vi "Lab Panel V4.87.vi"() -> ()   [LabVIEW 2013] (continued)
                      frame "CYCLE TEST" {
                      }
                      frame "T-RISE TEST" {
                      }
                    }
                    n1119 = Increment(x=w2157) -> (x+1=w2158:dbl)
                    n1120 = Greater Or Equal?(x=w2165, y=w2158) -> (x >= y?=w2167:bool)
                    n1121 = case shown="True" w2167 {
                      tunnel: w2162 -> [w2177 _]
                      tunnel: w2161 -> [w2176 _]
                      tunnel: w2160 -> [w2175 _]
                      tunnel: w2159 -> [w2174 _]
                      frame True {
                        n1122 = stacked-sequence {
                          tunnel: w2177 -> [w2181 _]
                          tunnel: w2176 -> [w2179 w2185]
                          tunnel: w2175 -> [_ w2188]
                          tunnel: w2174 -> [w2178 _]
                          frame #0 {
                            n1123 = Build Array(w2179) -> (w2182:string[])
                            n1124 = Build Array(w2181) -> (w2180:dbl[])
                            n1125 = TDMS Write(0:w2178, 5:"TEST PASS", 7:w2182, 9:w2180) -> (15:w2184:errorcluster)  [unwired: 2 in, 3 out]
                            n1126 = local write "data file error"(w2184) -> ()
                          }
                          frame #1 {
                            n1127 = Bundle(cluster=w2188, "STATUS"=w2185) -> (w2186:T4)  [unwired: 2 in]
                            n1128 = local write "RESULT LAB02-2"(TRUE) -> ()
                            n1129 = local write "DISP LAB02-2"(w2186) -> ()
                          }
                        }
                      }
                      frame False {
                      }
                    }
                  }
                }
              }
              frame #4 {
                # "LAB03-1"
                n1130 = Less?(x=w2189, y=2) -> (x < y?=w2192:bool)
                n1131 = local read "DISP LAB03-1"() -> (w2194:T4)
                n1132 = Unbundle(w2194) -> ("STATUS"=w2195:string)  [unwired: 2 out]
                n1133 = Equal?(x=w2195, y="RUN") -> (x = y?=w2191:bool)
                n1134 = And(x=w2191, y=w2192) -> (x .and. y?=w2190:bool)
                n1135 = case shown="True" w2190 {
                  tunnel: w2194 -> [_ w2200]
                  tunnel: w2189 -> [_ w2204]
                  frame False {
                  }
                  frame True {
                    n1136 = local read "SET LAB03-1"() -> (w2206:T5)
                    n1137 = local read "TDMS LAB03-1"() -> (w2199:refnum<k34>)
                    n1138 = Unbundle(w2200) -> ("CYCLE"=w2205:dbl)  [unwired: 2 out]
                    n1139 = Unbundle(w2206) -> ("CYCLES"=w2197:dbl, "T-RISE mins"=w2203:dbl)  [unwired: 3 out]
                    n1140 = case shown="\"T-RISE TEST\"" w2204 {
                      tunnel: w2203 -> [_ _ w2213]
                      tunnel: [w2208 w2210 w2213] -> w2202
                      tunnel: w2197 -> [w2208 w2210 _]
                      tunnel: ["CHART PASS" "CYCLE PASS" "T-RISE PASS"] -> w2201
                      frame "CHART TEST", Default {
                      }
                      frame "CYCLE TEST" {
                      }
                      frame "T-RISE TEST" {
                      }
                    }
                    n1141 = Increment(x=w2197) -> (x+1=w2198:dbl)
                    n1142 = Greater Or Equal?(x=w2205, y=w2198) -> (x >= y?=w2207:bool)
                    n1143 = case shown="True" w2207 {
                      tunnel: w2202 -> [w2217 _]
                      tunnel: w2201 -> [w2216 _]
                      tunnel: w2200 -> [w2215 _]
                      tunnel: w2199 -> [w2214 _]
                      frame True {
                        n1144 = stacked-sequence {
                          tunnel: w2217 -> [w2221 _]
                          tunnel: w2216 -> [w2219 w2225]
                          tunnel: w2215 -> [_ w2228]
                          tunnel: w2214 -> [w2218 _]
                          frame #0 {
                            n1145 = Build Array(w2219) -> (w2222:string[])
                            n1146 = Build Array(w2221) -> (w2220:dbl[])
                            n1147 = TDMS Write(0:w2218, 5:"TEST PASS", 7:w2222, 9:w2220) -> (15:w2224:errorcluster)  [unwired: 2 in, 3 out]
                            n1148 = local write "data file error"(w2224) -> ()
                          }
                          frame #1 {
                            n1149 = Bundle(cluster=w2228, "STATUS"=w2225) -> (w2226:T4)  [unwired: 2 in]
                            n1150 = local write "RESULT LAB03-1"(TRUE) -> ()
                            n1151 = local write "DISP LAB03-1"(w2226) -> ()
                          }
                        }
                      }
                      frame False {
                      }
                    }
                  }
                }
              }
              frame #5 {
                # "LAB03-2"
                n1152 = Less?(x=w2229, y=2) -> (x < y?=w2232:bool)
                n1153 = local read "DISP LAB03-2"() -> (w2234:T4)
                n1154 = Unbundle(w2234) -> ("STATUS"=w2235:string)  [unwired: 2 out]
                n1155 = Equal?(x=w2235, y="RUN") -> (x = y?=w2231:bool)
                n1156 = And(x=w2231, y=w2232) -> (x .and. y?=w2230:bool)
                n1157 = case shown="True" w2230 {
                  tunnel: w2234 -> [_ w2240]
                  tunnel: w2229 -> [_ w2244]
                  frame False {
                  }
                  frame True {
                    n1158 = local read "SET LAB03-2"() -> (w2246:T5)
                    n1159 = local read "TDMS LAB03-2"() -> (w2239:refnum<k34>)
                    n1160 = Unbundle(w2240) -> ("CYCLE"=w2245:dbl)  [unwired: 2 out]
                    n1161 = Unbundle(w2246) -> ("CYCLES"=w2237:dbl, "T-RISE mins"=w2243:dbl)  [unwired: 3 out]
                    n1162 = case shown="\"T-RISE TEST\"" w2244 {
                      tunnel: w2243 -> [_ _ w2253]
                      tunnel: [w2248 w2250 w2253] -> w2242
                      tunnel: w2237 -> [w2248 w2250 _]
                      tunnel: ["CHART PASS" "CYCLE PASS" "T-RISE PASS"] -> w2241
                      frame "CHART TEST", Default {
                      }
                      frame "CYCLE TEST" {
                      }
                      frame "T-RISE TEST" {
                      }
                    }
                    n1163 = Increment(x=w2237) -> (x+1=w2238:dbl)
                    n1164 = Greater Or Equal?(x=w2245, y=w2238) -> (x >= y?=w2247:bool)
                    n1165 = case shown="True" w2247 {
                      tunnel: w2242 -> [w2257 _]
                      tunnel: w2241 -> [w2256 _]
                      tunnel: w2240 -> [w2255 _]
                      tunnel: w2239 -> [w2254 _]
                      frame True {
                        n1166 = stacked-sequence {
                          tunnel: w2257 -> [w2261 _]
                          tunnel: w2256 -> [w2259 w2265]
                          tunnel: w2255 -> [_ w2268]
                          tunnel: w2254 -> [w2258 _]
                          frame #0 {
                            n1167 = Build Array(w2259) -> (w2262:string[])
                            n1168 = Build Array(w2261) -> (w2260:dbl[])
                            n1169 = TDMS Write(0:w2258, 5:"TEST PASS", 7:w2262, 9:w2260) -> (15:w2264:errorcluster)  [unwired: 2 in, 3 out]
                            n1170 = local write "data file error"(w2264) -> ()
                          }
                          frame #1 {
                            n1171 = Bundle(cluster=w2268, "STATUS"=w2265) -> (w2266:T4)  [unwired: 2 in]
                            n1172 = local write "RESULT LAB03-2"(TRUE) -> ()
                            n1173 = local write "DISP LAB03-2"(w2266) -> ()
                          }
                        }
                      }
                      frame False {
                      }
                    }
                  }
                }
              }
              frame #6 {
                # "LAB04-1"
                n1174 = Less?(x=w2269, y=2) -> (x < y?=w2272:bool)
                n1175 = local read "DISP LAB04-1"() -> (w2274:T4)
                n1176 = Unbundle(w2274) -> ("STATUS"=w2275:string)  [unwired: 2 out]
                n1177 = Equal?(x=w2275, y="RUN") -> (x = y?=w2271:bool)
                n1178 = And(x=w2271, y=w2272) -> (x .and. y?=w2270:bool)
                n1179 = case shown="True" w2270 {
                  tunnel: w2274 -> [_ w2280]
                  tunnel: w2269 -> [_ w2284]
                  frame False {
                  }
                  frame True {
                    n1180 = local read "SET LAB04-1"() -> (w2286:T5)
                    n1181 = local read "TDMS LAB04-1"() -> (w2279:refnum<k34>)
                    n1182 = Unbundle(w2280) -> ("CYCLE"=w2285:dbl)  [unwired: 2 out]
                    n1183 = Unbundle(w2286) -> ("CYCLES"=w2277:dbl, "T-RISE mins"=w2283:dbl)  [unwired: 3 out]
                    n1184 = case shown="\"T-RISE TEST\"" w2284 {
                      tunnel: w2283 -> [_ _ w2293]
                      tunnel: [w2288 w2290 w2293] -> w2282
                      tunnel: w2277 -> [w2288 w2290 _]
                      tunnel: ["CHART PASS" "CYCLE PASS" "T-RISE PASS"] -> w2281
                      frame "CHART TEST", Default {
                      }
                      frame "CYCLE TEST" {
                      }
                      frame "T-RISE TEST" {
                      }
                    }
                    n1185 = Increment(x=w2277) -> (x+1=w2278:dbl)
                    n1186 = Greater Or Equal?(x=w2285, y=w2278) -> (x >= y?=w2287:bool)
                    n1187 = case shown="True" w2287 {
                      tunnel: w2282 -> [w2297 _]
                      tunnel: w2281 -> [w2296 _]
                      tunnel: w2280 -> [w2295 _]
                      tunnel: w2279 -> [w2294 _]
                      frame True {
                        n1188 = stacked-sequence {
                          tunnel: w2297 -> [w2301 _]
                          tunnel: w2296 -> [w2299 w2305]
                          tunnel: w2295 -> [_ w2308]
                          tunnel: w2294 -> [w2298 _]
                          frame #0 {
                            n1189 = Build Array(w2299) -> (w2302:string[])
                            n1190 = Build Array(w2301) -> (w2300:dbl[])
                            n1191 = TDMS Write(0:w2298, 5:"TEST PASS", 7:w2302, 9:w2300) -> (15:w2304:errorcluster)  [unwired: 2 in, 3 out]
                            n1192 = local write "data file error"(w2304) -> ()
                          }
                          frame #1 {
                            n1193 = Bundle(cluster=w2308, "STATUS"=w2305) -> (w2306:T4)  [unwired: 2 in]
                            n1194 = local write "RESULT LAB04-1"(TRUE) -> ()
                            n1195 = local write "DISP LAB04-1"(w2306) -> ()
                          }
                        }
                      }
                      frame False {
                      }
                    }
                  }
                }
              }
              frame #7 {
                # "LAB04-2"
                n1196 = Less?(x=w2309, y=2) -> (x < y?=w2312:bool)
                n1197 = local read "DISP LAB04-2"() -> (w2314:T4)
                n1198 = Unbundle(w2314) -> ("STATUS"=w2315:string)  [unwired: 2 out]
                n1199 = Equal?(x=w2315, y="RUN") -> (x = y?=w2311:bool)
                n1200 = And(x=w2311, y=w2312) -> (x .and. y?=w2310:bool)
                n1201 = case shown="True" w2310 {
                  tunnel: w2314 -> [_ w2320]
                  tunnel: w2309 -> [_ w2324]
                  frame False {
                  }
                  frame True {
                    n1202 = local read "SET LAB04-2"() -> (w2326:T5)
                    n1203 = local read "TDMS LAB04-2"() -> (w2319:refnum<k34>)
                    n1204 = Unbundle(w2320) -> ("CYCLE"=w2325:dbl)  [unwired: 2 out]
                    n1205 = Unbundle(w2326) -> ("CYCLES"=w2317:dbl, "T-RISE mins"=w2323:dbl)  [unwired: 3 out]
                    n1206 = case shown="\"T-RISE TEST\"" w2324 {
                      tunnel: w2323 -> [_ _ w2333]
                      tunnel: [w2328 w2330 w2333] -> w2322
                      tunnel: w2317 -> [w2328 w2330 _]
                      tunnel: ["CHART PASS" "CYCLE PASS" "T-RISE PASS"] -> w2321
                      frame "CHART TEST", Default {
                      }
                      frame "CYCLE TEST" {
                      }
                      frame "T-RISE TEST" {
                      }
                    }
                    n1207 = Increment(x=w2317) -> (x+1=w2318:dbl)
                    n1208 = Greater Or Equal?(x=w2325, y=w2318) -> (x >= y?=w2327:bool)
                    n1209 = case shown="True" w2327 {
                      tunnel: w2322 -> [w2337 _]
                      tunnel: w2321 -> [w2336 _]
                      tunnel: w2320 -> [w2335 _]
                      tunnel: w2319 -> [w2334 _]
                      frame True {
                        n1210 = stacked-sequence {
                          tunnel: w2337 -> [w2341 _]
                          tunnel: w2336 -> [w2339 w2345]
                          tunnel: w2335 -> [_ w2348]
                          tunnel: w2334 -> [w2338 _]
                          frame #0 {
                            n1211 = Build Array(w2339) -> (w2342:string[])
                            n1212 = Build Array(w2341) -> (w2340:dbl[])
                            n1213 = TDMS Write(0:w2338, 5:"TEST PASS", 7:w2342, 9:w2340) -> (15:w2344:errorcluster)  [unwired: 2 in, 3 out]
                            n1214 = local write "data file error"(w2344) -> ()
                          }
                          frame #1 {
                            n1215 = Bundle(cluster=w2348, "STATUS"=w2345) -> (w2346:T4)  [unwired: 2 in]
                            n1216 = local write "RESULT LAB04-2"(TRUE) -> ()
                            n1217 = local write "DISP LAB04-2"(w2346) -> ()
                          }
                        }
                      }
                      frame False {
                      }
                    }
                  }
                }
              }
              frame #8 {
                # "LAB05-1"
                n1218 = Less?(x=w2349, y=2) -> (x < y?=w2352:bool)
                n1219 = local read "DISP LAB05-1"() -> (w2354:T4)
                n1220 = Unbundle(w2354) -> ("STATUS"=w2355:string)  [unwired: 2 out]
                n1221 = Equal?(x=w2355, y="RUN") -> (x = y?=w2351:bool)
                n1222 = And(x=w2351, y=w2352) -> (x .and. y?=w2350:bool)
                n1223 = case shown="True" w2350 {
                  tunnel: w2354 -> [_ w2360]
                  tunnel: w2349 -> [_ w2364]
                  frame False {
                  }
                  frame True {
                    n1224 = local read "SET LAB05-1"() -> (w2366:T5)
                    n1225 = local read "TDMS LAB05-1"() -> (w2359:refnum<k34>)
                    n1226 = Unbundle(w2360) -> ("CYCLE"=w2365:dbl)  [unwired: 2 out]
                    n1227 = Unbundle(w2366) -> ("CYCLES"=w2357:dbl, "T-RISE mins"=w2363:dbl)  [unwired: 3 out]
                    n1228 = case shown="\"T-RISE TEST\"" w2364 {
                      tunnel: w2363 -> [_ _ w2373]
                      tunnel: [w2368 w2370 w2373] -> w2362
                      tunnel: w2357 -> [w2368 w2370 _]
                      tunnel: ["CHART PASS" "CYCLE PASS" "T-RISE PASS"] -> w2361
                      frame "CHART TEST", Default {
                      }
                      frame "CYCLE TEST" {
                      }
                      frame "T-RISE TEST" {
                      }
                    }
                    n1229 = Increment(x=w2357) -> (x+1=w2358:dbl)
                    n1230 = Greater Or Equal?(x=w2365, y=w2358) -> (x >= y?=w2367:bool)
                    n1231 = case shown="True" w2367 {
                      tunnel: w2362 -> [w2377 _]
                      tunnel: w2361 -> [w2376 _]
                      tunnel: w2360 -> [w2375 _]
                      tunnel: w2359 -> [w2374 _]
                      frame True {
                        n1232 = stacked-sequence {
                          tunnel: w2377 -> [w2381 _]
                          tunnel: w2376 -> [w2379 w2385]
                          tunnel: w2375 -> [_ w2388]
                          tunnel: w2374 -> [w2378 _]
                          frame #0 {
                            n1233 = Build Array(w2379) -> (w2382:string[])
                            n1234 = Build Array(w2381) -> (w2380:dbl[])
                            n1235 = TDMS Write(0:w2378, 5:"TEST PASS", 7:w2382, 9:w2380) -> (15:w2384:errorcluster)  [unwired: 2 in, 3 out]
                            n1236 = local write "data file error"(w2384) -> ()
                          }
                          frame #1 {
                            n1237 = Bundle(cluster=w2388, "STATUS"=w2385) -> (w2386:T4)  [unwired: 2 in]
                            n1238 = local write "RESULT LAB05-1"(TRUE) -> ()
                            n1239 = local write "DISP LAB05-1"(w2386) -> ()
                          }
                        }
                      }
                      frame False {
                      }
                    }
                  }
                }
              }
              frame #9 {
                # "LAB05-2"
                n1240 = Less?(x=w2389, y=2) -> (x < y?=w2392:bool)
                n1241 = local read "DISP LAB05-2"() -> (w2394:T4)
                n1242 = Unbundle(w2394) -> ("STATUS"=w2395:string)  [unwired: 2 out]
                n1243 = Equal?(x=w2395, y="RUN") -> (x = y?=w2391:bool)
                n1244 = And(x=w2391, y=w2392) -> (x .and. y?=w2390:bool)
                n1245 = case shown="True" w2390 {
                  tunnel: w2394 -> [_ w2400]
                  tunnel: w2389 -> [_ w2404]
                  frame False {
                  }
                  frame True {
                    n1246 = local read "SET LAB05-2"() -> (w2406:T5)
                    n1247 = local read "TDMS LAB05-2"() -> (w2399:refnum<k34>)
                    n1248 = Unbundle(w2400) -> ("CYCLE"=w2405:dbl)  [unwired: 2 out]
                    n1249 = Unbundle(w2406) -> ("CYCLES"=w2397:dbl, "T-RISE mins"=w2403:dbl)  [unwired: 3 out]
                    n1250 = case shown="\"T-RISE TEST\"" w2404 {
                      tunnel: w2403 -> [_ _ w2413]
                      tunnel: [w2408 w2410 w2413] -> w2402
                      tunnel: w2397 -> [w2408 w2410 _]
                      tunnel: ["CHART PASS" "CYCLE PASS" "T-RISE PASS"] -> w2401
                      frame "CHART TEST", Default {
                      }
                      frame "CYCLE TEST" {
                      }
                      frame "T-RISE TEST" {
                      }
                    }
                    n1251 = Increment(x=w2397) -> (x+1=w2398:dbl)
                    n1252 = Greater Or Equal?(x=w2405, y=w2398) -> (x >= y?=w2407:bool)
                    n1253 = case shown="True" w2407 {
                      tunnel: w2402 -> [w2417 _]
                      tunnel: w2401 -> [w2416 _]
                      tunnel: w2400 -> [w2415 _]
                      tunnel: w2399 -> [w2414 _]
                      frame True {
                        n1254 = stacked-sequence {
                          tunnel: w2417 -> [w2421 _]
                          tunnel: w2416 -> [w2419 w2425]
                          tunnel: w2415 -> [_ w2428]
                          tunnel: w2414 -> [w2418 _]
                          frame #0 {
                            n1255 = Build Array(w2419) -> (w2422:string[])
                            n1256 = Build Array(w2421) -> (w2420:dbl[])
                            n1257 = TDMS Write(0:w2418, 5:"TEST PASS", 7:w2422, 9:w2420) -> (15:w2424:errorcluster)  [unwired: 2 in, 3 out]
                            n1258 = local write "data file error"(w2424) -> ()
                          }
                          frame #1 {
                            n1259 = Bundle(cluster=w2428, "STATUS"=w2425) -> (w2426:T4)  [unwired: 2 in]
                            n1260 = local write "RESULT LAB05-2"(TRUE) -> ()
                            n1261 = local write "DISP LAB05-2"(w2426) -> ()
                          }
                        }
                      }
                      frame False {
                      }
                    }
                  }
                }
              }
            }
          }
          frame #5 {
            # "check if test cycles reached for temperature rise test"
            n1262 = stacked-sequence {
              tunnel: w2458 -> [_ _ _ _ _ _ _ _ _ _]
              tunnel: w2457 -> [_ _ _ _ _ _ _ _ _ _]
              tunnel: w2456 -> [_ _ _ _ _ _ _ _ _ _]
              tunnel: w2455 -> [_ _ _ _ _ _ _ _ _ _]
              tunnel: w2454 -> [_ _ _ _ _ _ _ _ _ _]
              tunnel: w2453 -> [_ _ _ _ _ _ _ _ _ _]
              tunnel: w2452 -> [_ _ _ _ _ _ _ _ _ _]
              tunnel: w2451 -> [_ _ _ _ _ _ _ _ _ _]
              tunnel: w2450 -> [_ _ _ _ _ _ _ _ _ _]
              tunnel: w2449 -> [_ _ _ _ _ _ _ _ _ _]
              tunnel: w2448 -> [w2464 _ _ _ _ _ _ _ _ _]
              tunnel: w2438 -> [w2459 _ _ _ _ _ _ _ _ _]
              tunnel: w2447 -> [_ w2490 _ _ _ _ _ _ _ _]
              tunnel: w2446 -> [_ _ w2520 _ _ _ _ _ _ _]
              tunnel: w2445 -> [_ _ _ w2550 _ _ _ _ _ _]
              tunnel: w2444 -> [_ _ _ _ w2580 _ _ _ _ _]
              tunnel: w2443 -> [_ _ _ _ _ w2610 _ _ _ _]
              tunnel: w2442 -> [_ _ _ _ _ _ w2640 _ _ _]
              tunnel: w2441 -> [_ _ _ _ _ _ _ w2670 _ _]
              tunnel: w2440 -> [_ _ _ _ _ _ _ _ w2700 _]
              tunnel: w2439 -> [_ _ _ _ _ _ _ _ _ w2730]
              tunnel: w2437 -> [_ w2489 _ _ _ _ _ _ _ _]
              tunnel: w2436 -> [_ _ w2519 _ _ _ _ _ _ _]
              tunnel: w2435 -> [_ _ _ w2549 _ _ _ _ _ _]
              tunnel: w2434 -> [_ _ _ _ w2579 _ _ _ _ _]
              tunnel: w2433 -> [_ _ _ _ _ w2609 _ _ _ _]
              tunnel: w2432 -> [_ _ _ _ _ _ w2639 _ _ _]
              tunnel: w2431 -> [_ _ _ _ _ _ _ w2669 _ _]
              tunnel: w2430 -> [_ _ _ _ _ _ _ _ w2699 _]
              tunnel: w2429 -> [_ _ _ _ _ _ _ _ _ w2729]
              frame #0 {
                # "LAB01-1"
                n1263 = Equal?(x=w2464, y=2) -> (x = y?=w2462:bool)
                n1264 = local read "DISP LAB01-1"() -> (w2465:T4)
                n1265 = Unbundle(w2465) -> ("STATUS"=w2466:string)  [unwired: 2 out]
                n1266 = Equal?(x=w2466, y="RUN") -> (x = y?=w2461:bool)
                n1267 = And(x=w2461, y=w2462) -> (x .and. y?=w2460:bool)
                n1268 = case shown="True" w2460 {
                  tunnel: w2465 -> [_ w2469]
                  tunnel: w2459 -> [_ w2472]
                  frame False {
                  }
                  frame True {
                    n1269 = local read "SET LAB01-1"() -> (w2471:T5)
                    n1270 = local read "TDMS LAB01-1"() -> (w2468:refnum<k34>)
                    n1271 = Unbundle(w2469) -> ("CYCLE"=w2473:dbl)  [unwired: 2 out]
                    n1272 = Unbundle(w2471) -> ("T-RISE mins"=w2470:dbl)  [unwired: 4 out]
                    n1273 = Greater Or Equal?(x=w2473, y=w2472) -> (x >= y?=w2474:bool)
                    n1274 = case shown="True" w2474 {
                      tunnel: w2470 -> [w2477 _]
                      tunnel: w2469 -> [w2476 _]
                      tunnel: w2468 -> [w2475 _]
                      frame True {
                        n1275 = stacked-sequence {
                          tunnel: w2477 -> [w2480 _]
                          tunnel: w2476 -> [_ w2485]
                          tunnel: w2475 -> [w2478 _]
                          frame #0 {
                            n1276 = Build Array("T-RISE") -> (w2482:string[])
                            n1277 = Build Array(w2480) -> (w2481:dbl[])
                            n1278 = TDMS Write(0:w2478, 5:"TEST PASS", 7:w2482, 9:w2481) -> (15:w2484:errorcluster)  [unwired: 2 in, 3 out]
                            n1279 = local write "data file error"(w2484) -> ()
                          }
                          frame #1 {
                            n1280 = Bundle(cluster=w2485, "STATUS"="T-RISE PASS") -> (w2487:T4)  [unwired: 2 in]
                            n1281 = local write "RESULT LAB01-1"(TRUE) -> ()
                            n1282 = local write "DISP LAB01-1"(w2487) -> ()
                          }
                        }
                      }
                      frame False {
                      }
                    }
                  }
                }
              }
              frame #1 {
                # "LAB01-2"
                n1283 = Equal?(x=w2490, y=2) -> (x = y?=w2493:bool)
                n1284 = local read "DISP LAB01-2"() -> (w2495:T4)
                n1285 = Unbundle(w2495) -> ("STATUS"=w2496:string)  [unwired: 2 out]
                n1286 = Equal?(x=w2496, y="RUN") -> (x = y?=w2492:bool)
                n1287 = And(x=w2492, y=w2493) -> (x .and. y?=w2491:bool)
                n1288 = case shown="True" w2491 {
                  tunnel: w2495 -> [_ w2499]
                  tunnel: w2489 -> [_ w2502]
                  frame False {
                  }
                  frame True {
                    n1289 = local read "SET LAB01-2"() -> (w2501:T5)
                    n1290 = local read "TDMS LAB01-2"() -> (w2498:refnum<k34>)
                    n1291 = Unbundle(w2499) -> ("CYCLE"=w2503:dbl)  [unwired: 2 out]
                    n1292 = Unbundle(w2501) -> ("T-RISE mins"=w2500:dbl)  [unwired: 4 out]
                    n1293 = Greater Or Equal?(x=w2503, y=w2502) -> (x >= y?=w2504:bool)
                    n1294 = case shown="True" w2504 {
                      tunnel: w2500 -> [w2507 _]
                      tunnel: w2499 -> [w2506 _]
                      tunnel: w2498 -> [w2505 _]
                      frame True {
                        n1295 = stacked-sequence {
                          tunnel: w2507 -> [w2510 _]
                          tunnel: w2506 -> [_ w2515]
                          tunnel: w2505 -> [w2508 _]
                          frame #0 {
                            n1296 = Build Array("T-RISE") -> (w2512:string[])
                            n1297 = Build Array(w2510) -> (w2511:dbl[])
                            n1298 = TDMS Write(0:w2508, 5:"TEST PASS", 7:w2512, 9:w2511) -> (15:w2514:errorcluster)  [unwired: 2 in, 3 out]
                            n1299 = local write "data file error"(w2514) -> ()
                          }
                          frame #1 {
                            n1300 = Bundle(cluster=w2515, "STATUS"="T-RISE PASS") -> (w2517:T4)  [unwired: 2 in]
                            n1301 = local write "RESULT LAB01-2"(TRUE) -> ()
                            n1302 = local write "DISP LAB01-2"(w2517) -> ()
                          }
                        }
                      }
                      frame False {
                      }
                    }
                  }
                }
              }
              frame #2 {
                # "LAB02-1"
                n1303 = Equal?(x=w2520, y=2) -> (x = y?=w2523:bool)
                n1304 = local read "DISP LAB02-1"() -> (w2525:T4)
                n1305 = Unbundle(w2525) -> ("STATUS"=w2526:string)  [unwired: 2 out]
                n1306 = Equal?(x=w2526, y="RUN") -> (x = y?=w2522:bool)
                n1307 = And(x=w2522, y=w2523) -> (x .and. y?=w2521:bool)
                n1308 = case shown="True" w2521 {
                  tunnel: w2525 -> [_ w2529]
                  tunnel: w2519 -> [_ w2532]
                  frame False {
                  }
                  frame True {
                    n1309 = local read "SET LAB02-1"() -> (w2531:T5)
                    n1310 = local read "TDMS LAB02-1"() -> (w2528:refnum<k34>)
                    n1311 = Unbundle(w2529) -> ("CYCLE"=w2533:dbl)  [unwired: 2 out]
                    n1312 = Unbundle(w2531) -> ("T-RISE mins"=w2530:dbl)  [unwired: 4 out]
                    n1313 = Greater Or Equal?(x=w2533, y=w2532) -> (x >= y?=w2534:bool)
                    n1314 = case shown="True" w2534 {
                      tunnel: w2530 -> [w2537 _]
                      tunnel: w2529 -> [w2536 _]
                      tunnel: w2528 -> [w2535 _]
                      frame True {
                        n1315 = stacked-sequence {
                          tunnel: w2537 -> [w2540 _]
                          tunnel: w2536 -> [_ w2545]
                          tunnel: w2535 -> [w2538 _]
                          frame #0 {
                            n1316 = Build Array("T-RISE") -> (w2542:string[])
                            n1317 = Build Array(w2540) -> (w2541:dbl[])
                            n1318 = TDMS Write(0:w2538, 5:"TEST PASS", 7:w2542, 9:w2541) -> (15:w2544:errorcluster)  [unwired: 2 in, 3 out]
                            n1319 = local write "data file error"(w2544) -> ()
                          }
                          frame #1 {
                            n1320 = Bundle(cluster=w2545, "STATUS"="T-RISE PASS") -> (w2547:T4)  [unwired: 2 in]
                            n1321 = local write "RESULT LAB02-1"(TRUE) -> ()
                            n1322 = local write "DISP LAB02-1"(w2547) -> ()
                          }
                        }
                      }
                      frame False {
                      }
                    }
                  }
                }
              }
              frame #3 {
                # "LAB02-2"
                n1323 = Equal?(x=w2550, y=2) -> (x = y?=w2553:bool)
                n1324 = local read "DISP LAB02-2"() -> (w2555:T4)
                n1325 = Unbundle(w2555) -> ("STATUS"=w2556:string)  [unwired: 2 out]
                n1326 = Equal?(x=w2556, y="RUN") -> (x = y?=w2552:bool)
                n1327 = And(x=w2552, y=w2553) -> (x .and. y?=w2551:bool)
                n1328 = case shown="True" w2551 {
                  tunnel: w2555 -> [_ w2559]
                  tunnel: w2549 -> [_ w2562]
                  frame False {
                  }
                  frame True {
                    n1329 = local read "SET LAB02-2"() -> (w2561:T5)
                    n1330 = local read "TDMS LAB02-2"() -> (w2558:refnum<k34>)
                    n1331 = Unbundle(w2559) -> ("CYCLE"=w2563:dbl)  [unwired: 2 out]
                    n1332 = Unbundle(w2561) -> ("T-RISE mins"=w2560:dbl)  [unwired: 4 out]
                    n1333 = Greater Or Equal?(x=w2563, y=w2562) -> (x >= y?=w2564:bool)
                    n1334 = case shown="True" w2564 {
                      tunnel: w2560 -> [w2567 _]
                      tunnel: w2559 -> [w2566 _]
                      tunnel: w2558 -> [w2565 _]
                      frame True {
                        n1335 = stacked-sequence {
                          tunnel: w2567 -> [w2570 _]
                          tunnel: w2566 -> [_ w2575]
                          tunnel: w2565 -> [w2568 _]
                          frame #0 {
                            n1336 = Build Array("T-RISE") -> (w2572:string[])
                            n1337 = Build Array(w2570) -> (w2571:dbl[])
                            n1338 = TDMS Write(0:w2568, 5:"TEST PASS", 7:w2572, 9:w2571) -> (15:w2574:errorcluster)  [unwired: 2 in, 3 out]
                            n1339 = local write "data file error"(w2574) -> ()
                          }
                          frame #1 {
                            n1340 = Bundle(cluster=w2575, "STATUS"="T-RISE PASS") -> (w2577:T4)  [unwired: 2 in]
                            n1341 = local write "RESULT LAB02-2"(TRUE) -> ()
                            n1342 = local write "DISP LAB02-2"(w2577) -> ()
                          }
                        }
                      }
                      frame False {
                      }
                    }
                  }
                }
              }
              frame #4 {
                # "LAB03-1"
                n1343 = Equal?(x=w2580, y=2) -> (x = y?=w2583:bool)
                n1344 = local read "DISP LAB03-1"() -> (w2585:T4)
                n1345 = Unbundle(w2585) -> ("STATUS"=w2586:string)  [unwired: 2 out]
                n1346 = Equal?(x=w2586, y="RUN") -> (x = y?=w2582:bool)
                n1347 = And(x=w2582, y=w2583) -> (x .and. y?=w2581:bool)
                n1348 = case shown="True" w2581 {
                  tunnel: w2585 -> [_ w2589]
                  tunnel: w2579 -> [_ w2592]
                  frame False {
                  }
                  frame True {
                    n1349 = local read "SET LAB03-1"() -> (w2591:T5)
                    n1350 = local read "TDMS LAB03-1"() -> (w2588:refnum<k34>)
                    n1351 = Unbundle(w2589) -> ("CYCLE"=w2593:dbl)  [unwired: 2 out]
                    n1352 = Unbundle(w2591) -> ("T-RISE mins"=w2590:dbl)  [unwired: 4 out]
                    n1353 = Greater Or Equal?(x=w2593, y=w2592) -> (x >= y?=w2594:bool)
                    n1354 = case shown="True" w2594 {
                      tunnel: w2590 -> [w2597 _]
                      tunnel: w2589 -> [w2596 _]
                      tunnel: w2588 -> [w2595 _]
                      frame True {
                        n1355 = stacked-sequence {
                          tunnel: w2597 -> [w2600 _]
                          tunnel: w2596 -> [_ w2605]
                          tunnel: w2595 -> [w2598 _]
                          frame #0 {
                            n1356 = Build Array("T-RISE") -> (w2602:string[])
                            n1357 = Build Array(w2600) -> (w2601:dbl[])
                            n1358 = TDMS Write(0:w2598, 5:"TEST PASS", 7:w2602, 9:w2601) -> (15:w2604:errorcluster)  [unwired: 2 in, 3 out]
                            n1359 = local write "data file error"(w2604) -> ()
                          }
                          frame #1 {
                            n1360 = Bundle(cluster=w2605, "STATUS"="T-RISE PASS") -> (w2607:T4)  [unwired: 2 in]
                            n1361 = local write "RESULT LAB03-1"(TRUE) -> ()
                            n1362 = local write "DISP LAB03-1"(w2607) -> ()
                          }
                        }
                      }
                      frame False {
                      }
                    }
                  }
                }
              }
              frame #5 {
                # "LAB03-2"
                n1363 = Equal?(x=w2610, y=2) -> (x = y?=w2613:bool)
                n1364 = local read "DISP LAB03-2"() -> (w2615:T4)
                n1365 = Unbundle(w2615) -> ("STATUS"=w2616:string)  [unwired: 2 out]
                n1366 = Equal?(x=w2616, y="RUN") -> (x = y?=w2612:bool)
                n1367 = And(x=w2612, y=w2613) -> (x .and. y?=w2611:bool)
                n1368 = case shown="True" w2611 {
                  tunnel: w2615 -> [_ w2619]
                  tunnel: w2609 -> [_ w2622]
                  frame False {
                  }
                  frame True {
                    n1369 = local read "SET LAB03-2"() -> (w2621:T5)
                    n1370 = local read "TDMS LAB03-2"() -> (w2618:refnum<k34>)
                    n1371 = Unbundle(w2619) -> ("CYCLE"=w2623:dbl)  [unwired: 2 out]
                    n1372 = Unbundle(w2621) -> ("T-RISE mins"=w2620:dbl)  [unwired: 4 out]
                    n1373 = Greater Or Equal?(x=w2623, y=w2622) -> (x >= y?=w2624:bool)
                    n1374 = case shown="True" w2624 {
                      tunnel: w2620 -> [w2627 _]
                      tunnel: w2619 -> [w2626 _]
                      tunnel: w2618 -> [w2625 _]
                      frame True {
                        n1375 = stacked-sequence {
                          tunnel: w2627 -> [w2630 _]
                          tunnel: w2626 -> [_ w2635]
                          tunnel: w2625 -> [w2628 _]
                          frame #0 {
                            n1376 = Build Array("T-RISE") -> (w2632:string[])
                            n1377 = Build Array(w2630) -> (w2631:dbl[])
                            n1378 = TDMS Write(0:w2628, 5:"TEST PASS", 7:w2632, 9:w2631) -> (15:w2634:errorcluster)  [unwired: 2 in, 3 out]
                            n1379 = local write "data file error"(w2634) -> ()
                          }
                          frame #1 {
                            n1380 = Bundle(cluster=w2635, "STATUS"="T-RISE PASS") -> (w2637:T4)  [unwired: 2 in]
                            n1381 = local write "RESULT LAB03-2"(TRUE) -> ()
                            n1382 = local write "DISP LAB03-2"(w2637) -> ()
                          }
                        }
                      }
                      frame False {
                      }
                    }
                  }
                }
              }
              frame #6 {
                # "LAB04-1"
                n1383 = Equal?(x=w2640, y=2) -> (x = y?=w2643:bool)
                n1384 = local read "DISP LAB04-1"() -> (w2645:T4)
                n1385 = Unbundle(w2645) -> ("STATUS"=w2646:string)  [unwired: 2 out]
                n1386 = Equal?(x=w2646, y="RUN") -> (x = y?=w2642:bool)
                n1387 = And(x=w2642, y=w2643) -> (x .and. y?=w2641:bool)
                n1388 = case shown="True" w2641 {
                  tunnel: w2645 -> [_ w2649]
                  tunnel: w2639 -> [_ w2652]
                  frame False {
                  }
                  frame True {
                    n1389 = local read "SET LAB04-1"() -> (w2651:T5)
                    n1390 = local read "TDMS LAB04-1"() -> (w2648:refnum<k34>)
                    n1391 = Unbundle(w2649) -> ("CYCLE"=w2653:dbl)  [unwired: 2 out]
                    n1392 = Unbundle(w2651) -> ("T-RISE mins"=w2650:dbl)  [unwired: 4 out]
                    n1393 = Greater Or Equal?(x=w2653, y=w2652) -> (x >= y?=w2654:bool)
                    n1394 = case shown="True" w2654 {
                      tunnel: w2650 -> [w2657 _]
                      tunnel: w2649 -> [w2656 _]
                      tunnel: w2648 -> [w2655 _]
                      frame True {
                        n1395 = stacked-sequence {
                          tunnel: w2657 -> [w2660 _]
                          tunnel: w2656 -> [_ w2665]
                          tunnel: w2655 -> [w2658 _]
                          frame #0 {
                            n1396 = Build Array("T-RISE") -> (w2662:string[])
                            n1397 = Build Array(w2660) -> (w2661:dbl[])
                            n1398 = TDMS Write(0:w2658, 5:"TEST PASS", 7:w2662, 9:w2661) -> (15:w2664:errorcluster)  [unwired: 2 in, 3 out]
                            n1399 = local write "data file error"(w2664) -> ()
                          }
                          frame #1 {
                            n1400 = Bundle(cluster=w2665, "STATUS"="T-RISE PASS") -> (w2667:T4)  [unwired: 2 in]
                            n1401 = local write "RESULT LAB04-1"(TRUE) -> ()
                            n1402 = local write "DISP LAB04-1"(w2667) -> ()
                          }
                        }
                      }
                      frame False {
                      }
                    }
                  }
                }
              }
              frame #7 {
                # "LAB04-2"
                n1403 = Equal?(x=w2670, y=2) -> (x = y?=w2673:bool)
                n1404 = local read "DISP LAB04-2"() -> (w2675:T4)
                n1405 = Unbundle(w2675) -> ("STATUS"=w2676:string)  [unwired: 2 out]
                n1406 = Equal?(x=w2676, y="RUN") -> (x = y?=w2672:bool)
                n1407 = And(x=w2672, y=w2673) -> (x .and. y?=w2671:bool)
                n1408 = case shown="True" w2671 {
                  tunnel: w2675 -> [_ w2679]
                  tunnel: w2669 -> [_ w2682]
                  frame False {
                  }
                  frame True {
                    n1409 = local read "SET LAB04-2"() -> (w2681:T5)
                    n1410 = local read "TDMS LAB04-2"() -> (w2678:refnum<k34>)
                    n1411 = Unbundle(w2679) -> ("CYCLE"=w2683:dbl)  [unwired: 2 out]
                    n1412 = Unbundle(w2681) -> ("T-RISE mins"=w2680:dbl)  [unwired: 4 out]
                    n1413 = Greater Or Equal?(x=w2683, y=w2682) -> (x >= y?=w2684:bool)
                    n1414 = case shown="True" w2684 {
                      tunnel: w2680 -> [w2687 _]
                      tunnel: w2679 -> [w2686 _]
                      tunnel: w2678 -> [w2685 _]
                      frame True {
                        n1415 = stacked-sequence {
                          tunnel: w2687 -> [w2690 _]
                          tunnel: w2686 -> [_ w2695]
                          tunnel: w2685 -> [w2688 _]
                          frame #0 {
                            n1416 = Build Array("T-RISE") -> (w2692:string[])
                            n1417 = Build Array(w2690) -> (w2691:dbl[])
                            n1418 = TDMS Write(0:w2688, 5:"TEST PASS", 7:w2692, 9:w2691) -> (15:w2694:errorcluster)  [unwired: 2 in, 3 out]
                            n1419 = local write "data file error"(w2694) -> ()
                          }
                          frame #1 {
                            n1420 = Bundle(cluster=w2695, "STATUS"="T-RISE PASS") -> (w2697:T4)  [unwired: 2 in]
                            n1421 = local write "RESULT LAB04-2"(TRUE) -> ()
                            n1422 = local write "DISP LAB04-2"(w2697) -> ()
                          }
                        }
                      }
                      frame False {
                      }
                    }
                  }
                }
              }
              frame #8 {
                # "LAB05-1"
                n1423 = Equal?(x=w2700, y=2) -> (x = y?=w2703:bool)
                n1424 = local read "DISP LAB05-1"() -> (w2705:T4)
                n1425 = Unbundle(w2705) -> ("STATUS"=w2706:string)  [unwired: 2 out]
                n1426 = Equal?(x=w2706, y="RUN") -> (x = y?=w2702:bool)
                n1427 = And(x=w2702, y=w2703) -> (x .and. y?=w2701:bool)
                n1428 = case shown="True" w2701 {
                  tunnel: w2705 -> [_ w2709]
                  tunnel: w2699 -> [_ w2712]
                  frame False {
                  }
                  frame True {
                    n1429 = local read "SET LAB05-1"() -> (w2711:T5)
                    n1430 = local read "TDMS LAB05-1"() -> (w2708:refnum<k34>)
                    n1431 = Unbundle(w2709) -> ("CYCLE"=w2713:dbl)  [unwired: 2 out]
                    n1432 = Unbundle(w2711) -> ("T-RISE mins"=w2710:dbl)  [unwired: 4 out]
                    n1433 = Greater Or Equal?(x=w2713, y=w2712) -> (x >= y?=w2714:bool)
                    n1434 = case shown="True" w2714 {
                      tunnel: w2710 -> [w2717 _]
                      tunnel: w2709 -> [w2716 _]
                      tunnel: w2708 -> [w2715 _]
                      frame True {
                        n1435 = stacked-sequence {
                          tunnel: w2717 -> [w2720 _]
                          tunnel: w2716 -> [_ w2725]
                          tunnel: w2715 -> [w2718 _]
                          frame #0 {
                            n1436 = Build Array("T-RISE") -> (w2722:string[])
                            n1437 = Build Array(w2720) -> (w2721:dbl[])
                            n1438 = TDMS Write(0:w2718, 5:"TEST PASS", 7:w2722, 9:w2721) -> (15:w2724:errorcluster)  [unwired: 2 in, 3 out]
                            n1439 = local write "data file error"(w2724) -> ()
                          }
                          frame #1 {
                            n1440 = Bundle(cluster=w2725, "STATUS"="T-RISE PASS") -> (w2727:T4)  [unwired: 2 in]
                            n1441 = local write "RESULT LAB05-1"(TRUE) -> ()
                            n1442 = local write "DISP LAB05-1"(w2727) -> ()
                          }
                        }
                      }
                      frame False {
                      }
                    }
                  }
                }
              }
              frame #9 {
                # "LAB05-2"
                n1443 = Equal?(x=w2730, y=2) -> (x = y?=w2733:bool)
                n1444 = local read "DISP LAB05-2"() -> (w2735:T4)
                n1445 = Unbundle(w2735) -> ("STATUS"=w2736:string)  [unwired: 2 out]
                n1446 = Equal?(x=w2736, y="RUN") -> (x = y?=w2732:bool)
                n1447 = And(x=w2732, y=w2733) -> (x .and. y?=w2731:bool)
                n1448 = case shown="True" w2731 {
                  tunnel: w2735 -> [_ w2739]
                  tunnel: w2729 -> [_ w2742]
                  frame False {
                  }
                  frame True {
                    n1449 = local read "SET LAB05-2"() -> (w2741:T5)
                    n1450 = local read "TDMS LAB05-2"() -> (w2738:refnum<k34>)
                    n1451 = Unbundle(w2739) -> ("CYCLE"=w2743:dbl)  [unwired: 2 out]
                    n1452 = Unbundle(w2741) -> ("T-RISE mins"=w2740:dbl)  [unwired: 4 out]
                    n1453 = Greater Or Equal?(x=w2743, y=w2742) -> (x >= y?=w2744:bool)
                    n1454 = case shown="True" w2744 {
                      tunnel: w2740 -> [w2747 _]
                      tunnel: w2739 -> [w2746 _]
                      tunnel: w2738 -> [w2745 _]
                      frame True {
                        n1455 = stacked-sequence {
                          tunnel: w2747 -> [w2750 _]
                          tunnel: w2746 -> [_ w2755]
                          tunnel: w2745 -> [w2748 _]
                          frame #0 {
                            n1456 = Build Array("T-RISE") -> (w2752:string[])
                            n1457 = Build Array(w2750) -> (w2751:dbl[])
                            n1458 = TDMS Write(0:w2748, 5:"TEST PASS", 7:w2752, 9:w2751) -> (15:w2754:errorcluster)  [unwired: 2 in, 3 out]
                            n1459 = local write "data file error"(w2754) -> ()
                          }
                          frame #1 {
                            n1460 = Bundle(cluster=w2755, "STATUS"="T-RISE PASS") -> (w2757:T4)  [unwired: 2 in]
                            n1461 = local write "RESULT LAB05-2"(TRUE) -> ()
                            n1462 = local write "DISP LAB05-2"(w2757) -> ()
                          }
                        }
                      }
                      frame False {
                      }
                    }
                  }
                }
              }
            }
          }
          frame #6 {
            # "end test & close test files"
            n1463 = local read "MAIL SETTINGS"() -> (w2763:T7)
            n1464 = Unbundle(w2763) -> ("OUT SERVER ADDRESS"=w2762:string, "FROM ACCOUNT"=w2761:string)  [unwired: 5 out]
            n1465 = stacked-sequence {
              tunnel: w2773 -> [_ _ _ _ _ _ _ _ _ _]
              tunnel: w2774 -> [_ _ _ _ _ _ _ _ _ _]
              tunnel: w2772 -> [_ _ _ _ _ _ _ _ _ _]
              tunnel: w2771 -> [_ _ _ _ _ _ _ _ _ _]
              tunnel: w2770 -> [_ _ _ _ _ _ _ _ _ _]
              tunnel: w2769 -> [_ _ _ _ _ _ _ _ _ _]
              tunnel: w2768 -> [_ _ _ _ _ _ _ _ _ _]
              tunnel: w2767 -> [_ _ _ _ _ _ _ _ _ _]
              tunnel: w2766 -> [_ _ _ _ _ _ _ _ _ _]
              tunnel: w2765 -> [_ _ _ _ _ _ _ _ _ _]
              tunnel: w2762 -> [w2778 w2830 w2878 w2925 w2972 w3019 w3066 w3113 w3160 w3207]
              tunnel: w2761 -> [w2777 w2829 w2877 w2924 w2971 w3018 w3065 w3112 w3159 w3206]
              tunnel: "Mail Test File To:" -> [w2776 w2828 w2876 w2923 w2970 w3017 w3064 w3111 w3158 w3205]
              tunnel: "Mail Test Fail" -> [w2775 w2827 w2875 w2922 w2969 w3016 w3063 w3110 w3157 w3204]
              frame #0 {
                # "LAB01-1"
                n1466 = local read "DISP LAB01-1"() -> (w2782:T4)
                n1467 = local read "run lab01-1"() -> (w2779:bool)
                n1468 = local read "TDMS LAB01-1"() -> (w2780:refnum<k34>)
                n1469 = Unbundle(w2782) -> ("CYCLE"=w2783:dbl, "STATUS"=w2781:string)  [unwired: 1 out]
                n1470 = case shown="True" w2779 {
                  tunnel: w2783 -> [_ w2789]
                  tunnel: w2782 -> [_ w2791]
                  tunnel: w2781 -> [_ w2788]
                  tunnel: w2780 -> [_ w2790]
                  tunnel: w2778 -> [_ w2787]
                  tunnel: w2777 -> [_ w2786]
                  tunnel: w2776 -> [_ w2785]
                  tunnel: w2775 -> [_ w2784]
                  frame False {
                  }
                  frame True {
                    n1471 = Not Equal?(x=w2788, y="RUN") -> (x != y?=w2792:bool)
                    n1472 = Greater?(x=w2789, y=2.0) -> (0:w2794:bool)
                    n1473 = And(x=w2794, y=w2792) -> (x .and. y?=w2793:bool)
                    n1474 = case shown="True" w2793 {
                      tunnel: w2791 -> [_ w2804]
                      tunnel: w2790 -> [_ w2803]
                      tunnel: w2789 -> [_ w2802]
                      tunnel: w2788 -> [_ w2801]
                      tunnel: w2787 -> [_ w2800]
